vi "Laboratory_VI2.vi"() -> ()   [LabVIEW 2022 SP3]
panel:
  out "Minimum":dbl
  out "Maximum":dbl
  in  "Number of repetitions":i16
  in  "Multiple":dbl
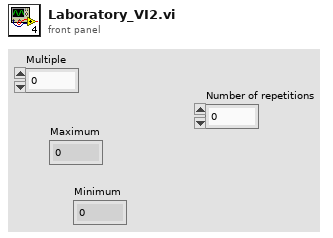
[diagram p1: front panel]
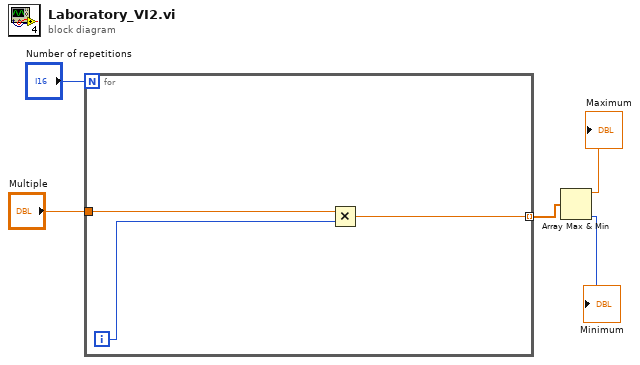
[diagram p0: block diagram]
diagram:
  n1 = for {
    N: "Number of repetitions" -> [_]
    tunnel: "Multiple" -> [w8]
    tunnel: [w6] -> w1 mode=indexing
    i -> [w7]
    n2 = Multiply(x=w8, y=w7) -> (x*y=w6:dbl)
  }
  n3 = Array Max & Min(array=w1) -> (max value=→"Maximum":dbl, min index (indices)=→"Minimum":i32)  [unwired: 2 out]
